vi "Test Context.vi"(8 "error in (no error)":errorcluster, 11 "RemoteControl.ZMQ in":refnum<class "RemoteControl.ZMQ.lvclass">) -> (0 "error out":errorcluster, 3 "RemoteControl.ZMQ out":refnum<class "RemoteControl.ZMQ.lvclass">)   [LabVIEW 2019]
uses:
  src/RemoteControl.ZMQ/RemoteControl.ZMQ.lvclass
  <vilib>/addons/zeromq/zmq_context.lvclass
  <vilib>/addons/_JKI Toolkits/Caraya/classes/Assert/Assert Not Error.vi
  <vilib>/addons/_JKI Toolkits/Caraya/classes/Assert/Assert Error.vi
  <vilib>/addons/_JKI Toolkits/Caraya/classes/Assert/Assert.lvclass
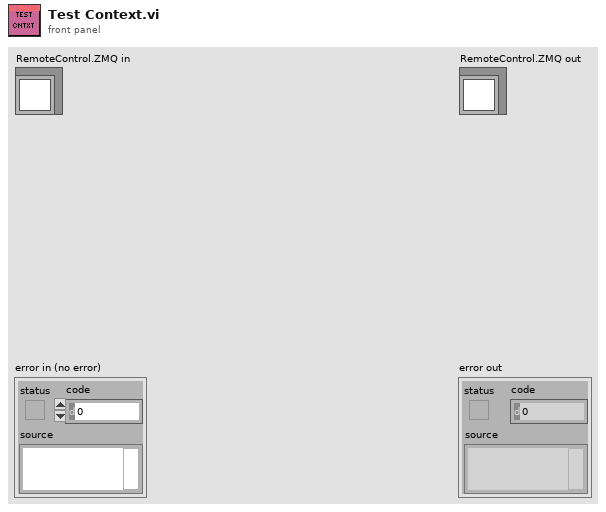
[diagram p1: front panel]
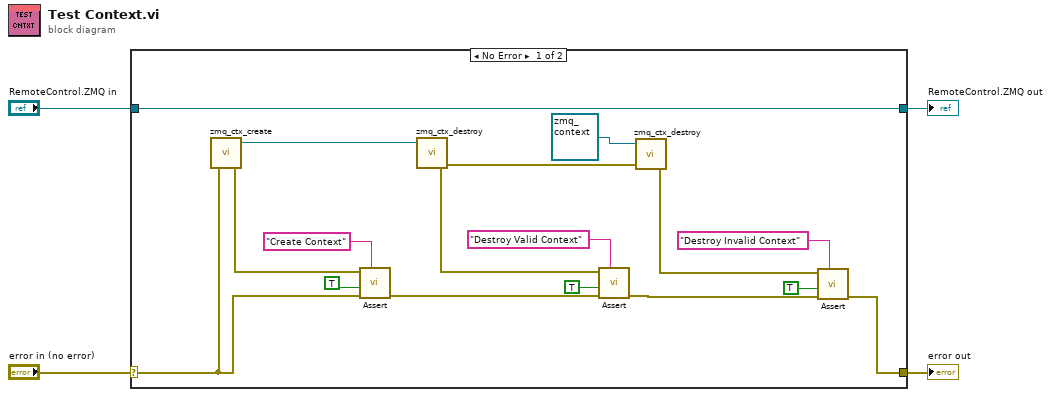
[diagram p0: block diagram]
diagram:
  n1 = case shown="No Error" "error in (no error)" {
    selector: "error in (no error)" -> [w18 w22]
    tunnel: [w5 w22] -> w3
    tunnel: [w16 w21] -> w1
    tunnel: "RemoteControl.ZMQ in" -> [w16 w21]
    frame No Error {
      n2 = call <vilib>:"zmq_ctx_create.vi"("error in"=w18) -> ("error out"=w20:errorcluster, "context out"=w12:refnum<class "zmq_context.lvclass">)  [unwired: 3 in]
      n3 = call-poly <vilib>:"Assert.vi"("Label"="Create Context", "error in (no error)"=w18, "Register with caller test (F)"=TRUE, "Not Error?"=w20) -> ("error out"=w13:errorcluster)  [unwired: 6 in, 1 out]
      n4 = call <vilib>:"zmq_ctx_destroy.vi"("context in"=w12) -> ("error out"=w6:errorcluster)  [unwired: 4 in]
      n5 = call-poly <vilib>:"Assert.vi"("Label"="Destroy Valid Context", "error in (no error)"=w13, "Register with caller test (F)"=TRUE, "Not Error?"=w6) -> ("error out"=w7:errorcluster)  [unwired: 6 in, 1 out]
      n6 = call <vilib>:"zmq_ctx_destroy.vi"("error in"=w6, "context in"=refnum<class "zmq_context.lvclass"> refnum) -> ("error out"=w8:errorcluster)  [unwired: 3 in]
      n7 = call-poly <vilib>:"Assert.vi"("Label"="Destroy Invalid Context", "error in (no error)"=w7, "Register with caller test (F)"=TRUE, "Error?"=w8) -> ("error out"=w5:errorcluster)  [unwired: 6 in, 1 out]
    }
    frame Error {
    }
  }
  "error out" <- w3
  "RemoteControl.ZMQ out" <- w1
